vi "SemanaIMonterreyExamen.vi"() -> ()   [LabVIEW 2018]
panel:
  out "Indicador Estado":T1(ring)
  out "Indicador Distancia Recorrida":i32
  in  "Control Salta":bool
  out "Indicador Dosis Disponibles":i32(slide) scale=0.0..20.0
  out "Indicador Zona Aleatoria":i32
  out "Indicador Zona":i32
  in  "Control Zona":i32(slide) scale=1.0..3.0
  out "Indicador Salud":i32(slide) caption="Indicador\n Salud" scale=0.0..10.0
  out "Indicador Nectar Tomado":i32(slide) caption="Indicador Nectar\n       Tomado" scale=0.0..5.0
  in  "Control Nectar":bool
  in  "stop":bool
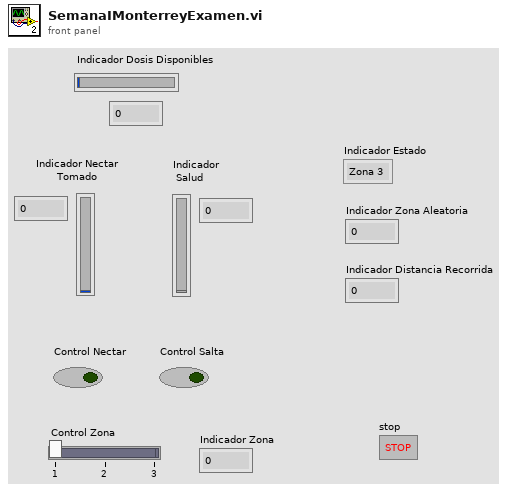
[diagram p1: front panel]
types:
  T1 = enum16{"Zona 3", "Zona 2", "Zona 1", "Volando", "Junta Nectar"}
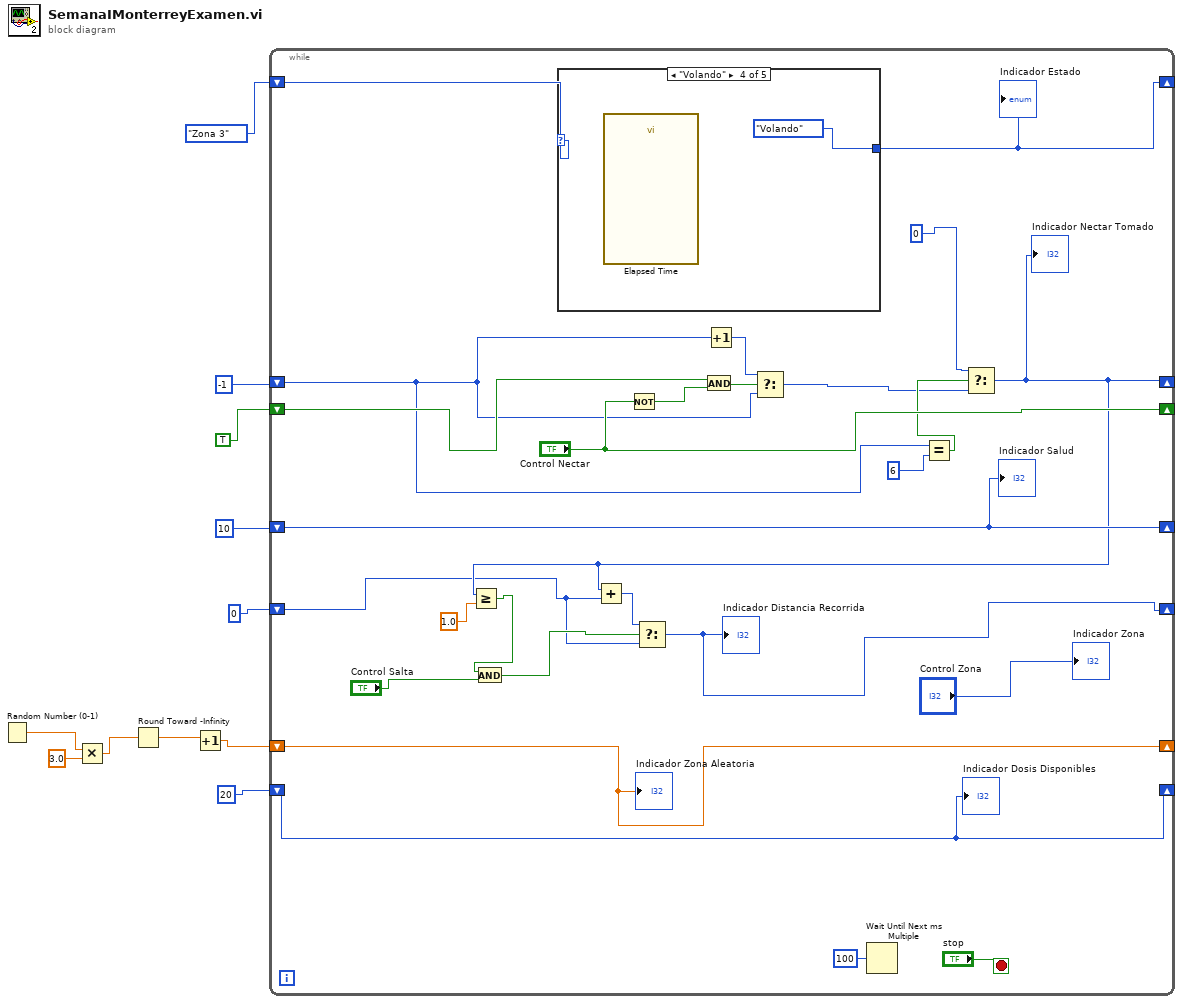
[diagram p0: block diagram]
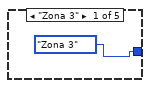
[diagram p2: hidden frame]
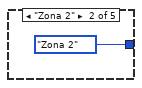
[diagram p3: hidden frame]
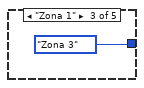
[diagram p4: hidden frame]
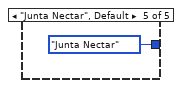
[diagram p5: hidden frame]
diagram:
  n1 = Random Number (0-1)() -> (number: 0 to 1=w6:dbl)
  n2 = Multiply(x=w6, y=3.0) -> (x*y=w7:dbl)
  n3 = Round Toward -Infinity(1:w7) -> (0:w8:dbl)
  n4 = Increment(x=w8) -> (x+1=w4:dbl)
  n5 = while {
    shift-right: [w14] -> _
    shift-left: -1 -> [w27]
    shift-right: ["Control Nectar"] -> _
    shift-left: TRUE -> [w32]
    shift-right: [w25] -> _
    shift-left: 10 -> [w25]
    shift-right: [w24] -> _
    shift-left: w4 -> [w24]
    shift-right: [w23] -> _
    shift-left: 20 -> [w23]
    shift-right: [w17] -> _
    shift-left: T1."Zona 3" -> [w22]
    shift-right: [w12] -> _
    shift-left: 0 -> [w13]
    stop <- "stop" stop-if-true
    n6 = case shown="\"Volando\"" w22 {
      tunnel: [T1."Zona 3" T1."Zona 2" T1."Zona 3" T1."Volando" T1."Junta Nectar"] -> w17
      frame "Zona 3" {
      }
      frame "Zona 2" {
      }
      frame "Zona 1" {
      }
      frame "Volando" {
        n7 = call "Elapsed Time"() -> ()  [unwired: 12 in, 8 out]
      }
      frame "Junta Nectar", Default {
      }
    }
    "Indicador Estado" <- w17
    n8 = Not(x="Control Nectar") -> (.not. x?=w35:bool)
    n9 = And(x=w32, y=w35) -> (x .and. y?=w34:bool)
    n10 = Increment(x=w27) -> (x+1=w33:i32)
    n11 = Select(t=w33, s=w34, f=w27) -> (s? t:f=w28:i32)
    n12 = Wait Until Next ms Multiple(millisecond multiple=u32 100) -> ()  [unwired: 1 out]
    n13 = Equal?(x=w27, y=6) -> (x = y?=w29:bool)
    n14 = Select(t=0, s=w29, f=w28) -> (s? t:f=w14:i32)
    "Indicador Nectar Tomado" <- w14
    n15 = Greater Or Equal?(x=w14, y=1.0) -> (x >= y?=w18:bool)
    n16 = And(x=w18, y="Control Salta") -> (x .and. y?=w16:bool)
    n17 = Add(x=w14, y=w13) -> (x+y=w15:i32)
    n18 = Select(t=w15, s=w16, f=w13) -> (s? t:f=w12:i32)
    "Indicador Distancia Recorrida" <- w12
    "Indicador Salud" <- w25
    "Indicador Zona" <- "Control Zona"
    "Indicador Zona Aleatoria" <- w24
    "Indicador Dosis Disponibles" <- w23
  }
